vi "Custom Tank.vi"(0 "RobotDriveDevRef 2":T8={"DevStatus"={"status"=FALSE, "code"=0, "source"=""}, "Motors[]"=[], "Square Inputs"=FALSE, "Max Output"=1.0}, 5 "Left axis value":dbl, 9 "Right axis value":dbl, 11 "error in (no error)":errorcluster) -> (4 "RobotDriveDevRef":T8={"DevStatus"={"status"=FALSE, "code"=0, "source"=""}, "Motors[]"=[], "Square Inputs"=FALSE, "Max Output"=1.0}, 6 "Middle Left Motor":T1={"DeviceStatus"={"status"=FALSE, "code"=0, "source"=""}, "Type"=enum."PWM", "PWM"={"PWM Channel"=enum."PWM 1", "DeadBand"={"Name"="", "maxPositivePwm"=0, "minPositivePwm"=0, "centerPwm"=0, "maxNegativePwm"=0, "minNegativePwm"=0, "angularRange"=0}}, "CAN"={"Device Number"=0, "Control Mode"=enum."Percent VBus", "Semaphore"=refnum, "Max Vout"=12.0, "TalonSRX Control Mode"=enum."Percent VBus"}, "Invert"=FALSE}, 8 "Middle Right Motor":T1={"DeviceStatus"={"status"=FALSE, "code"=0, "source"=""}, "Type"=enum."PWM", "PWM"={"PWM Channel"=enum."PWM 1", "DeadBand"={"Name"="", "maxPositivePwm"=0, "minPositivePwm"=0, "centerPwm"=0, "maxNegativePwm"=0, "minNegativePwm"=0, "angularRange"=0}}, "CAN"={"Device Number"=0, "Control Mode"=enum."Percent VBus", "Semaphore"=refnum, "Max Vout"=12.0, "TalonSRX Control Mode"=enum."Percent VBus"}, "Invert"=FALSE}, 10 "Motor Values":dbl[](array[numeric]), 15 "error out":errorcluster)   [LabVIEW 2015]
uses:
  <vilib>/Rock Robotics/WPI/RobotDrive/WPI_RobotDriveDevRef.ctl
  <vilib>/Rock Robotics/WPI/MotorControl/WPI_MotorControlDeviceRef.ctl
  <vilib>/Rock Robotics/WPI/MotorControl/WPI_MotorControlType.ctl
  <vilib>/Rock Robotics/SystemInterfaces/DIO/FPGA_DIOPWMChannel.ctl
  <vilib>/Rock Robotics/WPI/PWM/WPI_PWMDeadband.ctl
  <vilib>/Rock Robotics/WPI/CAN/Jaguar/SubVIs/WPI_CANJaguar_ControlMode.ctl
  <vilib>/Rock Robotics/WPI/CAN/TalonSRX/WPI_CANTalonSRX_APIControlMode.ctl
  <vilib>/Rock Robotics/SystemInterfaces/NetworkCommunication/NetComm_UsageReport_ResourceType.ctl
  Robot Global Data.vi
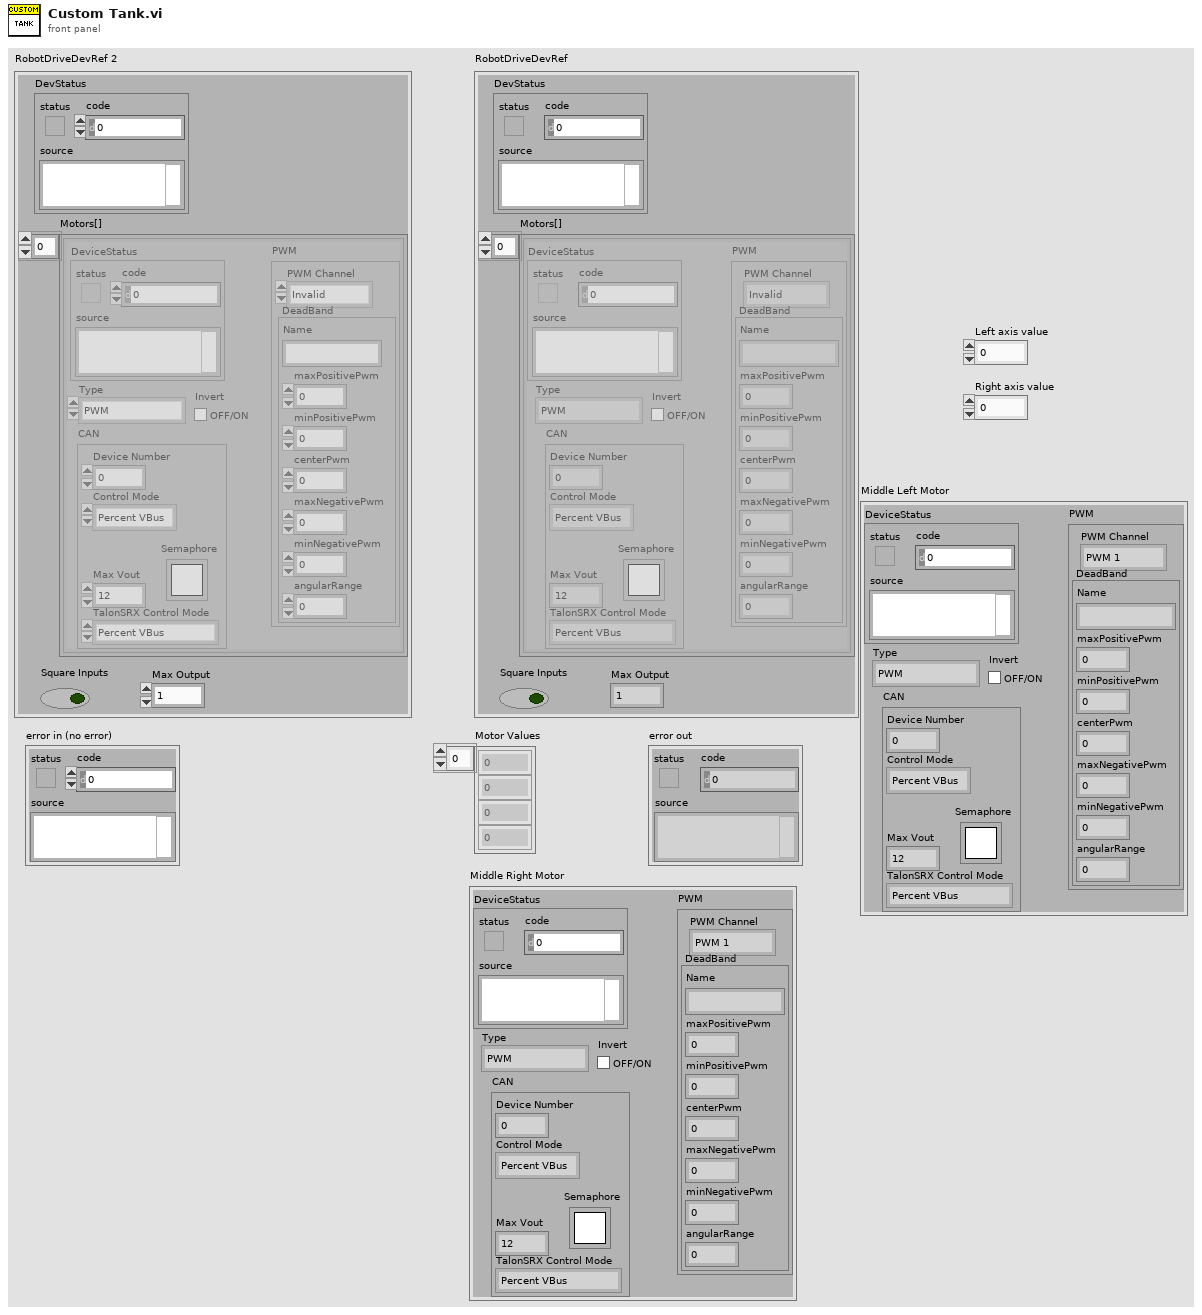
[diagram p1: front panel]
types:
  T1 = typedef "WPI_MotorControlDeviceRef.ctl" = cluster{"DeviceStatus":errorcluster, "Type":T2, "PWM":cluster{"PWM Channel":T3, "DeadBand":T4}, "CAN":cluster{"Device Number":u8, "Control Mode":T5, "Semaphore":T6, "Max Vout":dbl, "TalonSRX Control Mode":T7}, "Invert":bool}
  T2 = typedef "WPI_MotorControlType.ctl" = enum16{"PWM", "CAN", "CANTalonSRX"}
  T3 = typedef "FPGA_DIOPWMChannel.ctl" = enum8{"PWM 0", "PWM 1", "PWM 2", "PWM 3", "PWM 4", "PWM 5", "PWM 6", "PWM 7", "PWM 8", "PWM 9", "PWM MXP 0", "PWM MXP 1", "PWM MXP 2", "PWM MXP 3", "PWM MXP 4", "PWM MXP 5", "PWM MXP 6", "PWM MXP 7", "PWM MXP 8", "PWM MXP 9", "Invalid"}
  T4 = typedef "WPI_PWMDeadband.ctl" = cluster{"Name":string, "maxPositivePwm":i32, "minPositivePwm":i32, "centerPwm":i32, "maxNegativePwm":i32, "minNegativePwm":i32, "angularRange":u16}
  T5 = typedef "WPI_CANJaguar_ControlMode.ctl" = enum8{"Percent VBus", "Current", "Speed", "Position", "Voltage"}
  T6 = typedef "Semaphore RefNum" = refnum<k1>
  T7 = typedef "WPI_CANTalonSRX_APIControlMode.ctl" = enum8{"Percent VBus", "Speed", "Position", "Slave", "Unchanged / Invalid", "Voltage Compensation", "Current", "Motion Profile"}
  T8 = typedef "WPI_RobotDriveDevRef.ctl" = cluster{"DevStatus":errorcluster, "Motors[]":T1[], "Square Inputs":bool, "Max Output":dbl}
  T9 = typedef "NetComm_UsageReport_ResourceType.ctl" = enum8{"Controller", "Module", "Language", "CANPlugin", "Accelerometer", "ADXL345", "AnalogChannel", "AnalogTrigger", "AnalogTriggerOutput", "CANJaguar", "Compressor", "Counter", "Dashboard", "DigitalInput", "DigitalOutput", "DriverStationCIO", "DriverStationEIO", "DriverStationLCD", "Encoder", "GearTooth", "Gyro", "I2C", "Framework", "Jaguar", "Joystick", "Kinect", "KinectStick", "PIDController", "Preferences", "PWM", "Relay", "RobotDrive", "SerialPort", "Servo", "Solenoid", "SPI", "Task", "Ultrasonic", "Victor", "Button", "Command", "AxisCamera", "PCVideoServer", "SmartDashboard", "Talon", "HiTechnicColorSensor", "HiTechnicAccel", "HiTechnicCompass", "SRF08", "AnalogOutput", "Victor SP", "Talon SRX", "CAN Talon SRX", "ADXL362 Accel", "ADXRS450 Gyro", "Rev SPARK", "Mindsensors SD540", "Digital Filter"}
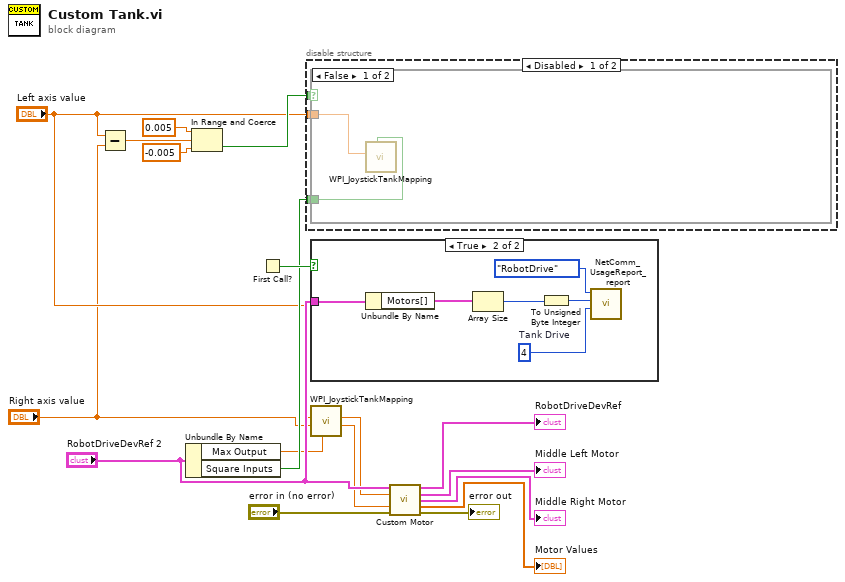
[diagram p0: block diagram]
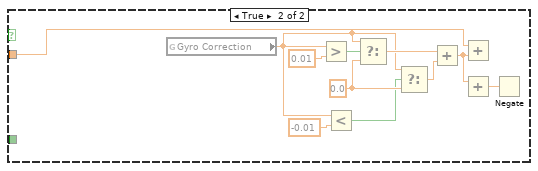
[diagram p2: hidden frame]
diagram:
  n1 = Subtract(x="Left axis value", y="Right axis value") -> (x-y=w9:dbl)
  n2 = Unbundle By Name("RobotDriveDevRef 2") -> ("Max Output"=w5:dbl, "Square Inputs"=w12:bool)
  n3 = In Range and Coerce(upper limit=0.005, x=w9, lower limit=-0.005) -> (In Range?=w6:bool)  [unwired: 1 out]
  n4 = First Call?() -> (First Call?: T/F=w18:bool)
  n5 = disable-structure shown="Disabled" {
    disable-tunnel: w12 -> [w21 _]
    disable-tunnel: "Left axis value" -> [w20 _]
    disable-tunnel: w6 -> [w19 _]
    frame Disabled {
      n6 = case shown="False" w19 {
        tunnel: w20 -> [w23 w28]
        tunnel: w21 -> [w22 _]
        frame False {
          n7 = call <vilib>:"WPI_JoystickTankMapping.vi"("Square Inputs"=w22, "Left axis value"=w23) -> ()  [unwired: 8 in, 2 out]
        }
        frame True {
          w35 = 0.0 ("f")
          n8 = global read "Robot Global Data.vi" "Gyro Correction"() -> (w24:dbl)
          n9 = Greater?(x=w24, y=0.01) -> (0:w33:bool)
          n10 = Less?(x=w24, y=-0.01) -> (x < y?=w34:bool)
          n11 = Select(t=w24, s=w33, f=w35) -> (s? t:f=w30:dbl)
          n12 = Select(t=w24, s=w34, f=w35) -> (s? t:f=w29:dbl)
          n13 = Add(x=w30, y=w29) -> (x+y=w27:dbl)
          n14 = Add(x=w28, y=w27) -> ()  [unwired: 1 out]
          n15 = Add(x=w27) -> (y=w26:dbl, x+y=w25:dbl)
          n16 = Negate(x=w25) -> ()  [unwired: 1 out]
        }
      }
    }
    frame Enabled {
    }
  }
  n17 = case shown="True" w18 {
    tunnel: "RobotDriveDevRef 2" -> [_ w36]
    frame False {
    }
    frame True {
      w39 = u8 4  # Tank Drive
      n18 = Unbundle By Name(w36) -> ("Motors[]"=w38:T1[])
      n19 = Array Size(array=w38) -> (size(s)=w37:i32)
      n20 = To Unsigned Byte Integer(number=w37) -> (unsigned 8bit integer=w40:u8)
      n21 = call <vilib>:"NetComm_UsageReport_report.vi"("Context"=w39, "Instance Number"=w40, "Resource Type"=NetComm_UsageReport_ResourceType."RobotDrive") -> ()  [unwired: 9 in]
    }
  }
  n22 = call <vilib>:"WPI_JoystickTankMapping.vi"("Max Output"=w5, "Right axis value"="Right axis value", "Left axis value"="Left axis value") -> ("Right Motor Value"=w3:dbl, "Left Motor Value"=w4:dbl)  [unwired: 7 in]
  n23 = call "Custom Motor.vi"("RobotDriveDevRef in"="RobotDriveDevRef 2", "LeftSpeed"=w4, "RightSpeed"=w3, "error in (no error)"="error in (no error)") -> ("RobotDriveDevRef out"=→"RobotDriveDevRef":T8, "Middle Left Motor"=→"Middle Left Motor":T1, "Middle Right Motor"=→"Middle Right Motor":T1, "Motor Values"=→"Motor Values":dbl[], "error out"=→"error out":errorcluster)  [unwired: 7 in]
